vi "Host_NetStreams.vi"() -> ()   [LabVIEW 2019]
panel:
  in  "Freq":dbl=1.0
  out "error out":errorcluster
  out "Sine":dbl[](graph)
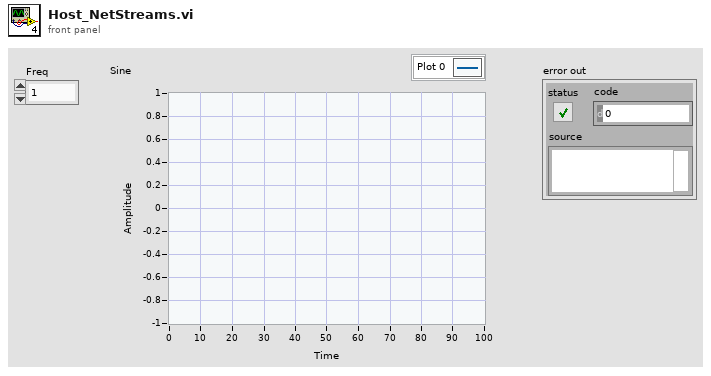
[diagram p1: front panel]
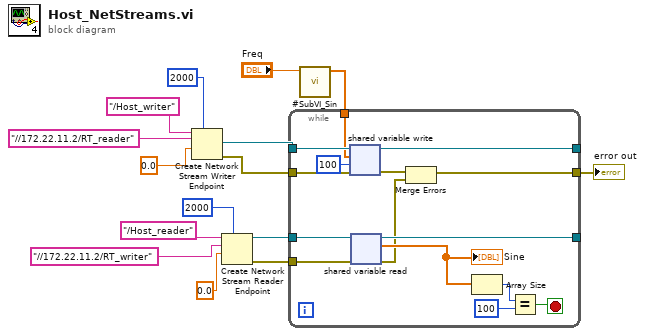
[diagram p0: block diagram]
diagram:
  n1 = Create Network Stream Writer Endpoint(7:2000 ("writer buffer size"), 9:0.0, 10:"//172.22.11.2/RT_reader" ("reader url"), 11:"/Host_writer" ("writer name")) -> (0:w4:errorcluster, 3:w5:refnum<k21>)  [unwired: 3 in]
  n2 = Create Network Stream Reader Endpoint(7:2000 ("reader buffer size"), 9:0.0, 10:"//172.22.11.2/RT_writer" ("reader url"), 11:"/Host_reader" ("reader name")) -> (0:w6:errorcluster, 3:w7:refnum<k21>)  [unwired: 3 in]
  n3 = call "#SubVI_Sin.vi"("Freq"="Freq") -> ("Waveform Graph"=w1:dbl[])  [unwired: 10 in]
  n4 = while {
    tunnel: w7 -> [w30]
    tunnel: w6 -> [w29]
    tunnel: w5 -> [w28]
    tunnel: w4 -> [w27]
    tunnel: [w26] -> _
    tunnel: [w18] -> w3
    tunnel: [w25] -> _
    tunnel: w1 -> [w23]
    stop <- w22 stop-if-true
    n5 = shared-variable-write(w28, w27, w23, 100 ("timeout ms (-1)")) -> (w26:refnum<k21>, w17:errorcluster)  [unwired: 1 out]
    n6 = shared-variable-read(w30, w29) -> (w25:refnum<k21>, w16:errorcluster, w19:dbl[])  [unwired: 2 in, 1 out]
    "Sine" <- w19
    n7 = Merge Errors(w17, w16) -> (w18:errorcluster)
    n8 = Array Size(array=w19) -> (size(s)=w21:i32)
    n9 = Equal?(x=w21, y=100) -> (x = y?=w22:bool)
  }
  "error out" <- w3
